vi "Test.vi"(7 "Label (VI Title)":string, 8 "error in (no error)":errorcluster, 11 "Type":variant) -> (0 "error out":errorcluster)   [LabVIEW 2018, in "JSON to LVConstant Test.lvlib"]
uses:
  JSON to LVConstant Test.lvlib
  9a1572e7-135a-41bf-ab18-c450e40867d5.vi
  <vilib>/JDP Science/JSONtext/Variant to JSON Text.vi
  <vilib>/addons/_JKI Toolkits/Caraya/classes/Assert/Assert Equal Type_Variant.vi
  <vilib>/addons/_JKI Toolkits/Caraya/classes/Assert/Assert Equal Value_Variant.vi
  <vilib>/JDP Science/JSONtext/LVClass Serializer/JSONtext LVClass Serializer.lvclass
  Source/SLL Scripting/SLL Scripting.lvlib
  <vilib>/addons/_JKI Toolkits/Caraya/classes/Assert/Assert.lvclass
  <vilib>/addons/_JKI Toolkits/Caraya/classes/Test/Test.lvclass
  <vilib>/JDP Science/JSONtext/JSONtext.lvlib
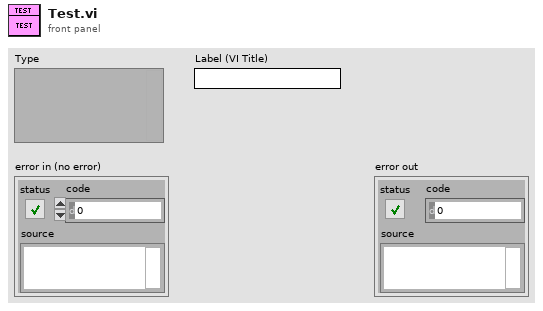
[diagram p1: front panel]
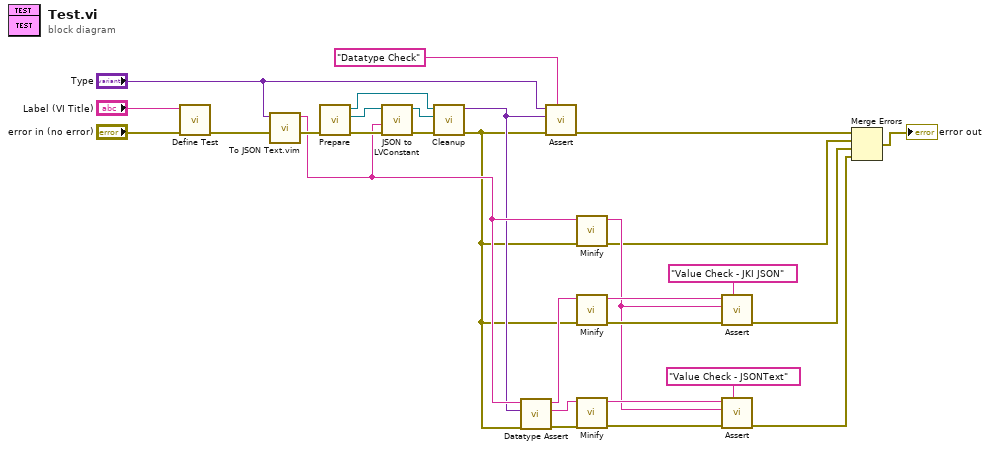
[diagram p0: block diagram]
diagram:
  n1 = call <vilib>:"Define Test.vi"("error in (no error)"="error in (no error)", "Label (VI Title)"="Label (VI Title)") -> ("error out"=w20:errorcluster)  [unwired: 9 in]
  n2 = call "To JSON Text.vim"("error in (no error)"=w20, "Anything"="Type") -> ("error out"=w25:errorcluster, "<JSON>"=w17:string)  [unwired: 8 in]
  n3 = call "Prepare.vi"("error in (no error)"=w25) -> ("error out"=w24:errorcluster, "Owner"=w26:refnum<vi>, "vi refnum"=w27:refnum<vi>)  [unwired: 8 in]
  n4 = call "JSON to LVConstant.vi"("error in (no error)"=w24, "<JSON>"=w17, "owner refnum in"=w26) -> ("error out"=w23:errorcluster, "owner refnum out"=w28:refnum<vi>)  [unwired: 7 in]
  n5 = call "Cleanup.vi"("error in (no error)"=w23, "Owner"=w28, "vi refnum"=w27) -> ("error out"=w11:errorcluster, "Type out"=w14:variant)  [unwired: 7 in]
  n6 = call "Datatype Assert.vi"("error in (no error)"=w11, "Data Type"=w14, "JSON"=w17) -> ("error out"=w12:errorcluster, "JSONText (Assert)"=w13:string, "JKIJSON (Assert)"=w16:string)  [unwired: 5 in, 1 out]
  n7 = call-poly <vilib>:"Assert.vi"("Label"="Datatype Check" ("Label (VI Title)"), "error in (no error)"=w11, "Y"=w14, "X"="Type") -> ("error out"=w29:errorcluster)  [unwired: 7 in]
  n8 = call <vilib>:"Minify.vi"("error in (no error)"=w11, "JSON"=w17) -> ("error out"=w1:errorcluster, "<JSON>"=w6:string)  [unwired: 7 in, 1 out]
  n9 = call <vilib>:"Minify.vi"("error in (no error)"=w11, "JSON"=w16) -> ("error out"=w8:errorcluster, "<JSON>"=w7:string)  [unwired: 7 in, 1 out]
  n10 = call <vilib>:"Minify.vi"("error in (no error)"=w12, "JSON"=w13) -> ("error out"=w10:errorcluster, "<JSON>"=w9:string)  [unwired: 7 in, 1 out]
  n11 = call-poly <vilib>:"Assert.vi"("Label"="Value Check - JKI JSON" ("Label (VI Title)"), "error in (no error)"=w8, "Y"=w6, "X"=w7) -> ("error out"=w5:errorcluster)  [unwired: 7 in]
  n12 = call-poly <vilib>:"Assert.vi"("Label"="Value Check - JSONText" ("Label (VI Title)"), "error in (no error)"=w10, "Y"=w6, "X"=w9) -> ("error out"=w4:errorcluster)  [unwired: 7 in]
  n13 = Merge Errors(w29, w1, w5, w4) -> (→"error out":errorcluster)
